vi "CommonVIs_FindBooleansInArray.vi"(1 "1D array":bool[](array[boolean]), 2 "element":bool=TRUE) -> (15 "index of element":i32, 16 "ArrayOfIndexOfElement":i32[](array[numeric]))   [LabVIEW 2016]
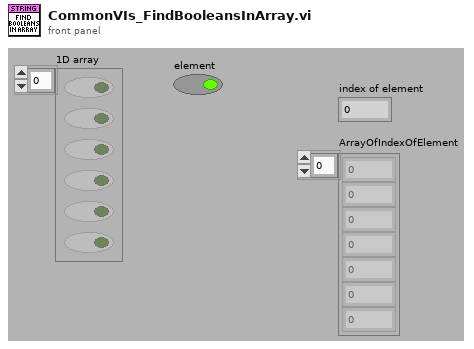
[diagram p1: front panel]
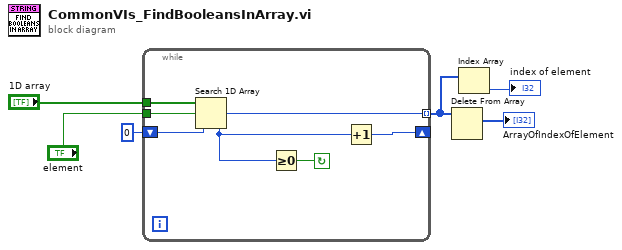
[diagram p0: block diagram]
diagram:
  n1 = while {
    tunnel: "element" -> [w12]
    tunnel: "1D array" -> [w11]
    shift-right: [w7] -> _
    shift-left: 0 ("index of element") -> [w10]
    tunnel: [w8] -> w3 mode=indexing
    stop <- w9 continue-if-true
    n2 = Search 1D Array(1D array=w11, element=w12, start index (0)=w10) -> (index of element=w8:i32)
    n3 = Greater Or Equal To 0?(x=w8) -> (x >= 0?=w9:bool)
    n4 = Increment(x=w8) -> (x+1=w7:i32)
  }
  n5 = Delete From Array(array=w3) -> (array with subset deleted=→"ArrayOfIndexOfElement":i32[])  [unwired: 2 in, 1 out]
  n6 = Index Array(array=w3) -> (element=→"index of element":i32)  [unwired: 1 in]
